vi "wa32 CreateNamedPipeA.vi"(5 "defaultTimeout (256k)":u32=256000, 7 "inBufferSize (256k)":u32=256000, 8 "error in":errorcluster, 9 "pipe mode":enum16{"Wait Mode", "No Wait Mode"}(ring), 10 "open mode":enum16{"INBOUND", "OUTBOUND", "DUPLEX"}(ring), 11 "file path":string="\\\\.\\Pipe\\MyNamedPipe") -> (0 "error out":errorcluster, 3 "handle":i32)   [LabVIEW 2020]
doc: "Wrapper for CreateFileA(). Opens or creates handle to files, devices, pipes, ... Don't forget to close the handle by CloseHandle()."
uses:
  <vilib>/Utility/error.llb/Error Cluster From Error Code.vi
  <vilib>/ErrorRing/Error Ring.xnode
  kernel32.dll
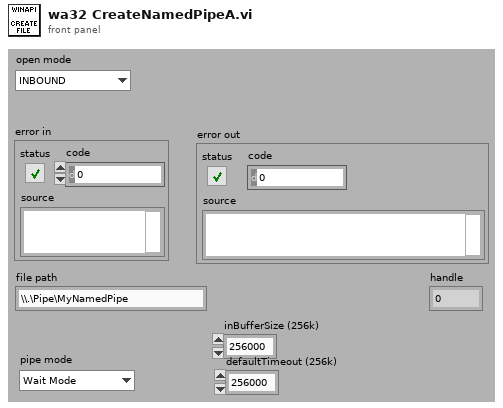
[diagram p1: front panel]
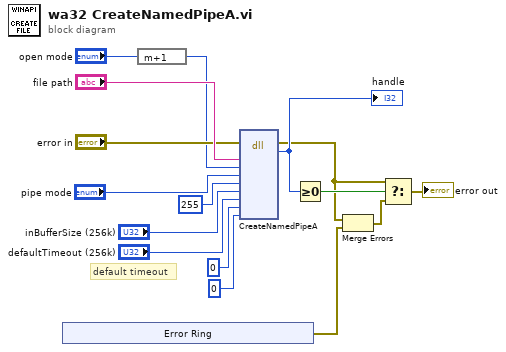
[diagram p0: block diagram]
diagram:
  # "default timeout"
  n1 = xnode "Error Ring"() -> ("error out"=w10:errorcluster)
  n2 = expression code="m+1"("open mode") -> (w2:enum16{"INBOUND", "OUTBOUND", "DUPLEX"})
  n3 = dll-call lib="kernel32.dll" fn="CreateNamedPipeA"(error in="error in", "name"="file path", "openMode"=w2, "pipeMode"="pipe mode", "maxInstances"=u32 255 ("outBufferSize"), "outBufferSize"="inBufferSize (256k)", "inBufferSize"="defaultTimeout (256k)", "defaultTimeout"=u32 0, "secAttributes"=0) -> (error out=w11:errorcluster, "handle"=w14:i32)  [unwired: 10 in, 1 out]
  "handle" <- w14
  n4 = Greater Or Equal To 0?(x=w14) -> (x >= 0?=w13:bool)
  n5 = Merge Errors(w11, w10) -> (w12:errorcluster)
  n6 = Select(t=w11, s=w13, f=w12) -> (s? t:f=→"error out":errorcluster)
